vi "LVInterface.vi"() -> ()   [LabVIEW 2017]
uses:
  <vilib>/httpClient/POSTBuffer.vi
  <vilib>/httpClient/LabVIEWHTTPClient.lvlib
panel:
  out "output cluster":cluster{"headers":string, "body":string}
  out "Array":cluster{"headers":string, "body":string}[](array[cluster])
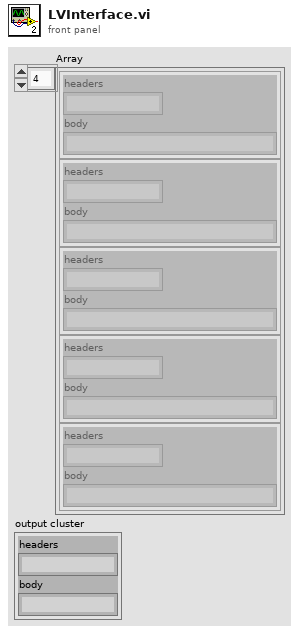
[diagram p1: front panel]
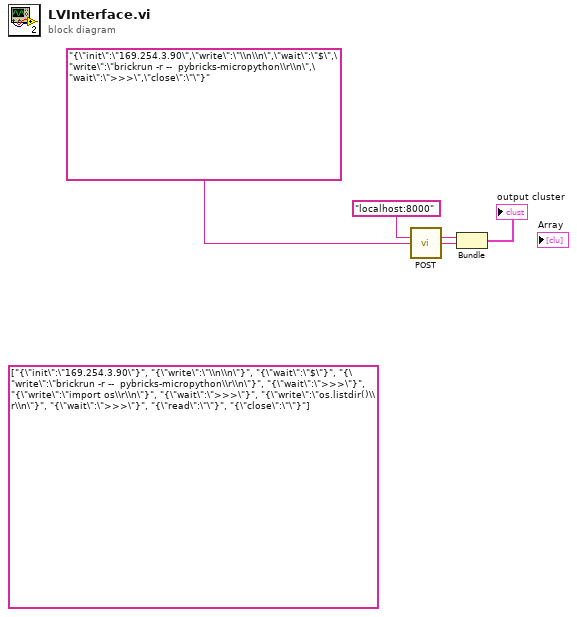
[diagram p0: block diagram]
diagram:
  (unwired) string[] ["{\"init\":\"169.254.3.90\"}", "{\"write\":\"\\n\\n\"}", "{\"wait\":\"$\"}", "{\"write\":\"brickrun -r --  pybricks-micropython\\r\\n\"}", "{\"wait\":\">>>\"}", "{\"write\":\"import os\\r\\n\"}", "{\"wait\":\">>>\"}", "{\"write\":\"os.listdir()\\r\\n\"}", "{\"wait\":\">>>\"}", "{\"read\":\"\"}", "{\"close\":\"\"}"]
  n1 = call-poly <vilib>:"POST.vi"("url"="localhost:8000", "buffer"="{\"init\":\"169.254.3.90\",\"write\":\"\\n\\n\",\"wait\":\"$\",\"write\":\"brickrun -r --  pybricks-micropython\\r\\n\",\"wait\":\">>>\",\"close\":\"\"}") -> ("headers"=w4:string, "body"=w3:string)  [unwired: 10 in, 2 out]
  n2 = Bundle("headers"=w4, "body"=w3) -> (→"output cluster":cluster{"headers":string, "body":string})  [unwired: 1 in]
